vi "pulse optimization panel.vi"() -> ()   [LabVIEW 2017]
panel:
  out "pulse analysis":T1
  out "pulse statistics":T2
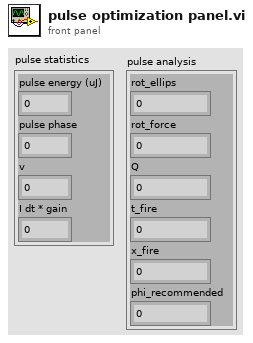
[diagram p1: front panel]
types:
  T1 = cluster{"rot_ellips":dbl, "rot_force":dbl, "Q":dbl, "t_fire":dbl, "x_fire":dbl, "phi_recommended":dbl}
  T2 = cluster{"pulse energy (uJ)":sgl, "pulse phase":dbl, "v":dbl, "I dt * gain":dbl}
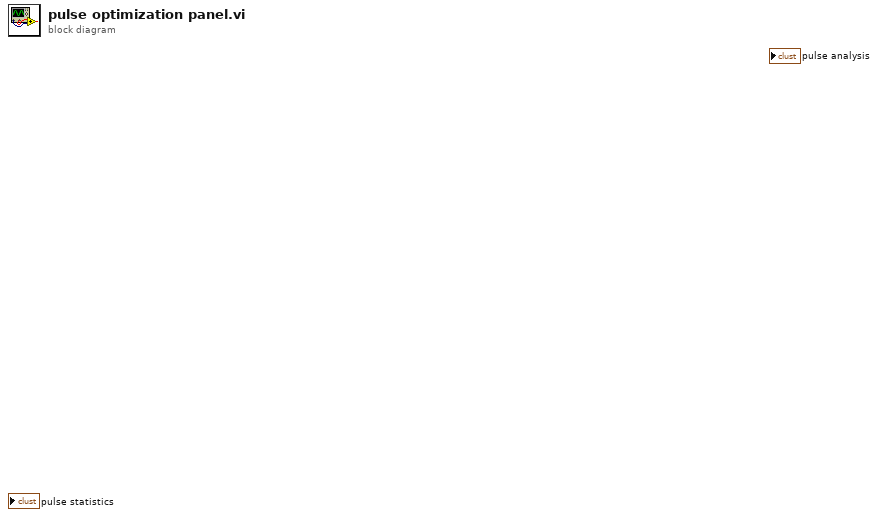
[diagram p0: block diagram]
diagram:
